vi "Set Initialized State.vi"(8 "error in (no error)":errorcluster, 10 "initialized":bool, 11 "motor communication in":refnum<class "NI_Robotics_Motor Communication.lvclass">) -> (0 "error out":errorcluster, 3 "motor communication out":refnum<class "NI_Robotics_Motor Communication.lvclass">)   [LabVIEW 2017, in "NI_Robotics_Motor Communication.lvclass"]
uses:
  <vilib>/robotics/Actuation/Motor Communication/NI_Robotics_Motor Communication.lvclass
  <vilib>/robotics/Actuation/Motor Communication/NI_Robotics_Motor Communication.lvclass/NI_Robotics_Motor Communication.ctl
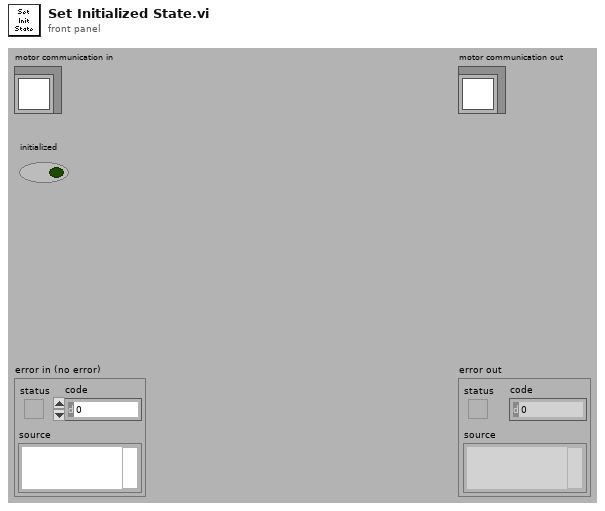
[diagram p1: front panel]
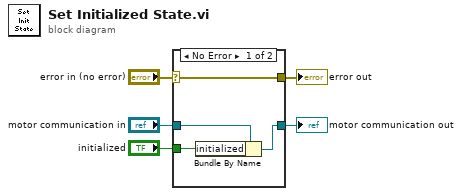
[diagram p0: block diagram]
diagram:
  n1 = case shown="No Error" "error in (no error)" {
    selector: "error in (no error)" -> [w9 w10]
    tunnel: [w9 w10] -> w4
    tunnel: [w7 w11] -> w2
    tunnel: "motor communication in" -> [w8 w11]
    tunnel: "initialized" -> [w6 _]
    frame No Error {
      n2 = Bundle By Name(cluster=w8, "initialized"=w6) -> (w7:refnum<class "NI_Robotics_Motor Communication.lvclass">)
    }
    frame Error {
    }
  }
  "error out" <- w4
  "motor communication out" <- w2
